vi "CTRE_Phoenix_MotorControl_ConfigureAllSettings.vi"(6 "timeoutMs":i32=50, 7 "Force Write":bool, 8 "error in (no error)":errorcluster, 10 "Motor Controller Configurables":T1={"Base Configurables"={"openLoopRamp"=0.0, "closedLoopRamp"=0.0, "peakOutputForward"=1.0, "peakOutputReverse"=-1.0, "nominalOutputForward"=0.0, "nominalOutputReverse"=0.0, "neutralDeadband"=0.04, "voltageCompSaturation"=0.0, "voltageMeasurementFilter"=32, "velocityMeasurementPeriod"=100, "velocityMeasurementWindow"=64, "forwardSoftLimitThreshold"=0, "reverseSoftLimitThreshold"=0, "forwardSoftLimitEnable"=FALSE, "reverseSoftLimitEnable"=FALSE, "slot0"={"P"=0.0, "I"=0.0, "D"=0.0, "F"=0.0, "integralZone"=0.0, "allowableClosedLoopError"=0, "maxIntegralAccumulator"=0.0, "closedLoopPeakOutput"=1.0, "closedLoopPeriod"=1}, "slot1"={"P"=0.0, "I"=0.0, "D"=0.0, "F"=0.0, "integralZone"=0.0, "allowableClosedLoopError"=0, "maxIntegralAccumulator"=0.0, "closedLoopPeakOutput"=1.0, "closedLoopPeriod"=1}, "slot2"={"P"=0.0, "I"=0.0, "D"=0.0, "F"=0.0, "integralZone"=0.0, "allowableClosedLoopError"=0, "maxIntegralAccumulator"=0.0, "closedLoopPeakOutput"=1.0, "closedLoopPeriod"=1}, "slot3"={"P"=0.0, "I"=0.0, "D"=0.0, "F"=0.0, "integralZone"=0.0, "allowableClosedLoopError"=0, "maxIntegralAccumulator"=0.0, "closedLoopPeakOutput"=1.0, "closedLoopPeriod"=1}, "auxPIDPolarity"=FALSE, "remoteFilter0"={"remoteSensorDeviceID"=0, "remoteSensorSource"=enum."Off"}, "remoteFilter1"={"remoteSensorDeviceID"=0, "remoteSensorSource"=enum."Off"}, "motionCruiseVelocity"=0, "motionAcceleration"=0, "motionProfileTrajectoryPeriod"=0, "feedbackNotContinuous"=FALSE, "remoteSensorClosedLoopDisableNeutralOnLOS"=FALSE, "clearPositionOnLimitF"=FALSE, "clearPositionOnLimitR"=FALSE, "clearPositionOnQuadIdx"=FALSE, "limitSwitchDisableNeutralOnLOS"=FALSE, "softLimitDisableNeutralOnLOS"=FALSE, "pulseWidthPeriod_EdgesPerRot"=1, "pulseWidthPeriod_FilterWindowSz"=1, "customParam"={"customParam0"=0, "customParam1"=0}, "trajectoryInterpolationEnable"=TRUE}, "primaryPID"={"selectedFeedbackCoefficient"=1.0, "selectedFeedbackSensor"=11}, "auxiliaryPID"={"selectedFeedbackCoefficient"=1.0, "selectedFeedbackSensor"=11}, "sum 0 term"=11, "sum 1 term"=11, "diff 0 term "=11, "diff 1 term"=11, "forwardLimitSwitchDeviceID"=0, "reverseLimitSwitchDeviceID"=0, "forwardLimitSwitchNormal"=enum."Normally Open", "reverseLimitSwitchNormal"=enum."Normally Open", "forwardLimitSwitchSource"=3, "reverseLimitSwitchSource"=3} {"diff 1 term" items=["Remote Source 0"=11, "Remote Source 1"=12, "Software Emulated"=15]; "diff 0 term" items=["Remote Source 0"=11, "Remote Source 1"=12, "Software Emulated"=15]; "sum 1 term" items=["Remote Source 0"=11, "Remote Source 1"=12, "Software Emulated"=15]; "sum 0 term" items=["Remote Source 0"=11, "Remote Source 1"=12, "Software Emulated"=15]; "reverseLimitSwitchSource" items=["Remote Talon SRX"=1, "Remote CANifier"=2, "Deactivated"=3]; "forwardLimitSwitchSource" items=["Remote Talon SRX"=1, "Remote CANifier"=2, "Deactivated"=3]; "auxiliaryPID"."selectedFeedbackSensor" items=["Sensor Sum (S0 + S1)"=9, "Sensor Difference (D0 - D1)"=10, "Remote Source 0"=11, "Remote Source 1"=12, "Software Emulated"=15]; "primaryPID"."selectedFeedbackSensor" items=["Sensor Sum (S0 + S1)"=9, "Sensor Difference (D0 - D1)"=10, "Remote Source 0"=11, "Remote Source 1"=12, "Software Emulated"=15]; "Base Configurables"."velocityMeasurementPeriod" items=["Period_1ms"=1, "Period_2ms"=2, "Period_5ms"=5, "Period_10ms"=10, "Period_20ms"=20, "Period_25ms"=25, "Period_50ms"=50, "Period_100ms"=100]}, 11 "PhoenixMotorControlDevRef":T12={"DeviceStatus"={"status"=FALSE, "code"=0, "source"=""}, "Type"=enum."PWM", "PWM"={"PWM Channel"=enum."PWM 1", "DeadBand"={"Name"="", "maxPositivePwm"=0, "minPositivePwm"=0, "centerPwm"=0, "maxNegativePwm"=0, "minNegativePwm"=0, "angularRange"=0}}, "CAN"={"Device Number"=0, "SetOutput VI Ref"=variant(enum8{"Percent VBus", "Current", "Speed", "Position", "Voltage"} enum."Percent VBus"), "GetOutput VI Ref"=variant(refnum<k1> refnum), "Enable VI Ref"=variant(dbl 12.0), "Disable VI Ref"=variant(enum8{"Percent VBus", "Speed", "Position", "Slave", "Unchanged / Invalid", "Voltage Compensation", "Current", "Motion Profile"} enum."Percent VBus"), "Data"=variant}, "Invert"=FALSE, "DIO PWM"={"PWM \"Enable\" Channel"=enum."Invalid", "DIOChannel"=enum."Invalid", "PWM Rate"=0.0}}) -> (0 "error out":errorcluster, 3 "PhoenixMotorControlDevRef":T12={"DeviceStatus"={"status"=FALSE, "code"=0, "source"=""}, "Type"=enum."PWM", "PWM"={"PWM Channel"=enum."PWM 1", "DeadBand"={"Name"="", "maxPositivePwm"=0, "minPositivePwm"=0, "centerPwm"=0, "maxNegativePwm"=0, "minNegativePwm"=0, "angularRange"=0}}, "CAN"={"Device Number"=0, "SetOutput VI Ref"=variant(enum8{"Percent VBus", "Current", "Speed", "Position", "Voltage"} enum."Percent VBus"), "GetOutput VI Ref"=variant(refnum<k1> refnum), "Enable VI Ref"=variant(dbl 12.0), "Disable VI Ref"=variant(enum8{"Percent VBus", "Speed", "Position", "Slave", "Unchanged / Invalid", "Voltage Compensation", "Current", "Motion Profile"} enum."Percent VBus"), "Data"=variant}, "Invert"=FALSE, "DIO PWM"={"PWM \"Enable\" Channel"=enum."Invalid", "DIOChannel"=enum."Invalid", "PWM Rate"=0.0}})   [LabVIEW 2020]
doc: "Configures all persistant settings\n\n<b> Motor Controller Configurables </b> Cluster of all items to be configured"
uses:
  <vilib>/Rock Robotics/WPI/MotorControl/WPI_MotorControlDeviceRef.ctl
  <vilib>/Rock Robotics/WPI/MotorControl/WPI_MotorControlType.ctl
  <vilib>/Rock Robotics/SystemInterfaces/DIO/FPGA_DIOPWMChannel.ctl
  <vilib>/Rock Robotics/WPI/PWM/WPI_PWMDeadband.ctl
  <vilib>/Rock Robotics/SystemInterfaces/DIO/FPGA_DIOChannel.ctl
  <vilib>/Rock Robotics/WPI/ThirdParty/Phoenix-LabVIEW/Motor Controller/Controls/CTRE_Phoenix_MotorControl_MotorControllerConfigurables.ctl
  <vilib>/Rock Robotics/WPI/ThirdParty/Phoenix-LabVIEW/Motor Controller/Controls/CTRE_Phoenix_MotorControl_BaseConfigurables.ctl
  <vilib>/Rock Robotics/WPI/ThirdParty/Phoenix-LabVIEW/Motor Controller/Controls/CTRE_Phoenix_MotorControl_VelocityMeasurementPeriod.ctl
  <vilib>/Rock Robotics/WPI/ThirdParty/Phoenix-LabVIEW/Motor Controller/Controls/CTRE_Phoenix_MotorControl_SlotStructure.ctl
  <vilib>/Rock Robotics/WPI/ThirdParty/Phoenix-LabVIEW/Motor Controller/Controls/CTRE_Phoenix_MotorControl_FilterStruct.ctl
  <vilib>/Rock Robotics/WPI/ThirdParty/Phoenix-LabVIEW/Motor Controller/Controls/CTRE_Phoenix_MotorControl_RemoteSourceType.ctl
  <vilib>/Rock Robotics/WPI/ThirdParty/Phoenix-LabVIEW/Controls/CTRE_Phoenix_CustomParamConfiguration.ctl
  <vilib>/Rock Robotics/WPI/ThirdParty/Phoenix-LabVIEW/Motor Controller/Controls/CTRE_Phoenix_MotorControl_RemoteFeedbackDevice.ctl
  <vilib>/Rock Robotics/WPI/ThirdParty/Phoenix-LabVIEW/Motor Controller/Controls/CTRE_Phoenix_MotorControl_SensorTermFeedbackDevice.ctl
  <vilib>/Rock Robotics/WPI/ThirdParty/Phoenix-LabVIEW/Motor Controller/Controls/CTRE_Phoenix_MotorControl_LimitSwitchNormal.ctl
  <vilib>/Rock Robotics/WPI/ThirdParty/Phoenix-LabVIEW/Motor Controller/Controls/CTRE_Phoenix_MotorControl_LimitSwitchSource.ctl
panel:
  # "Sum and Diff terms are ways to select more than one sensor as a feedback device. \n Sum 0 is the first feedback device to be used for the Sum term, \n Sum 1 is the feedback device to be added to Sum 0 for the Sum term\n Diff 0 and Diff 1 work in a similar manner"
  # "These are only applicable\nif using a remote limit switch.\n\nLocal limit switches/no limit\nswitches do not use this"
  # "False: Primary Output = PID[0] + PID[1]  ---  Auxiliary Output = PID[0] - PID[1]\nTrue:  Primary Output = PID[0] - PID[1] --- Auxiliary Output = PID[0] + PID[1]"
  # "Enable the motion profile executor to perform linear interpolation between profile points.  Defaults to True."
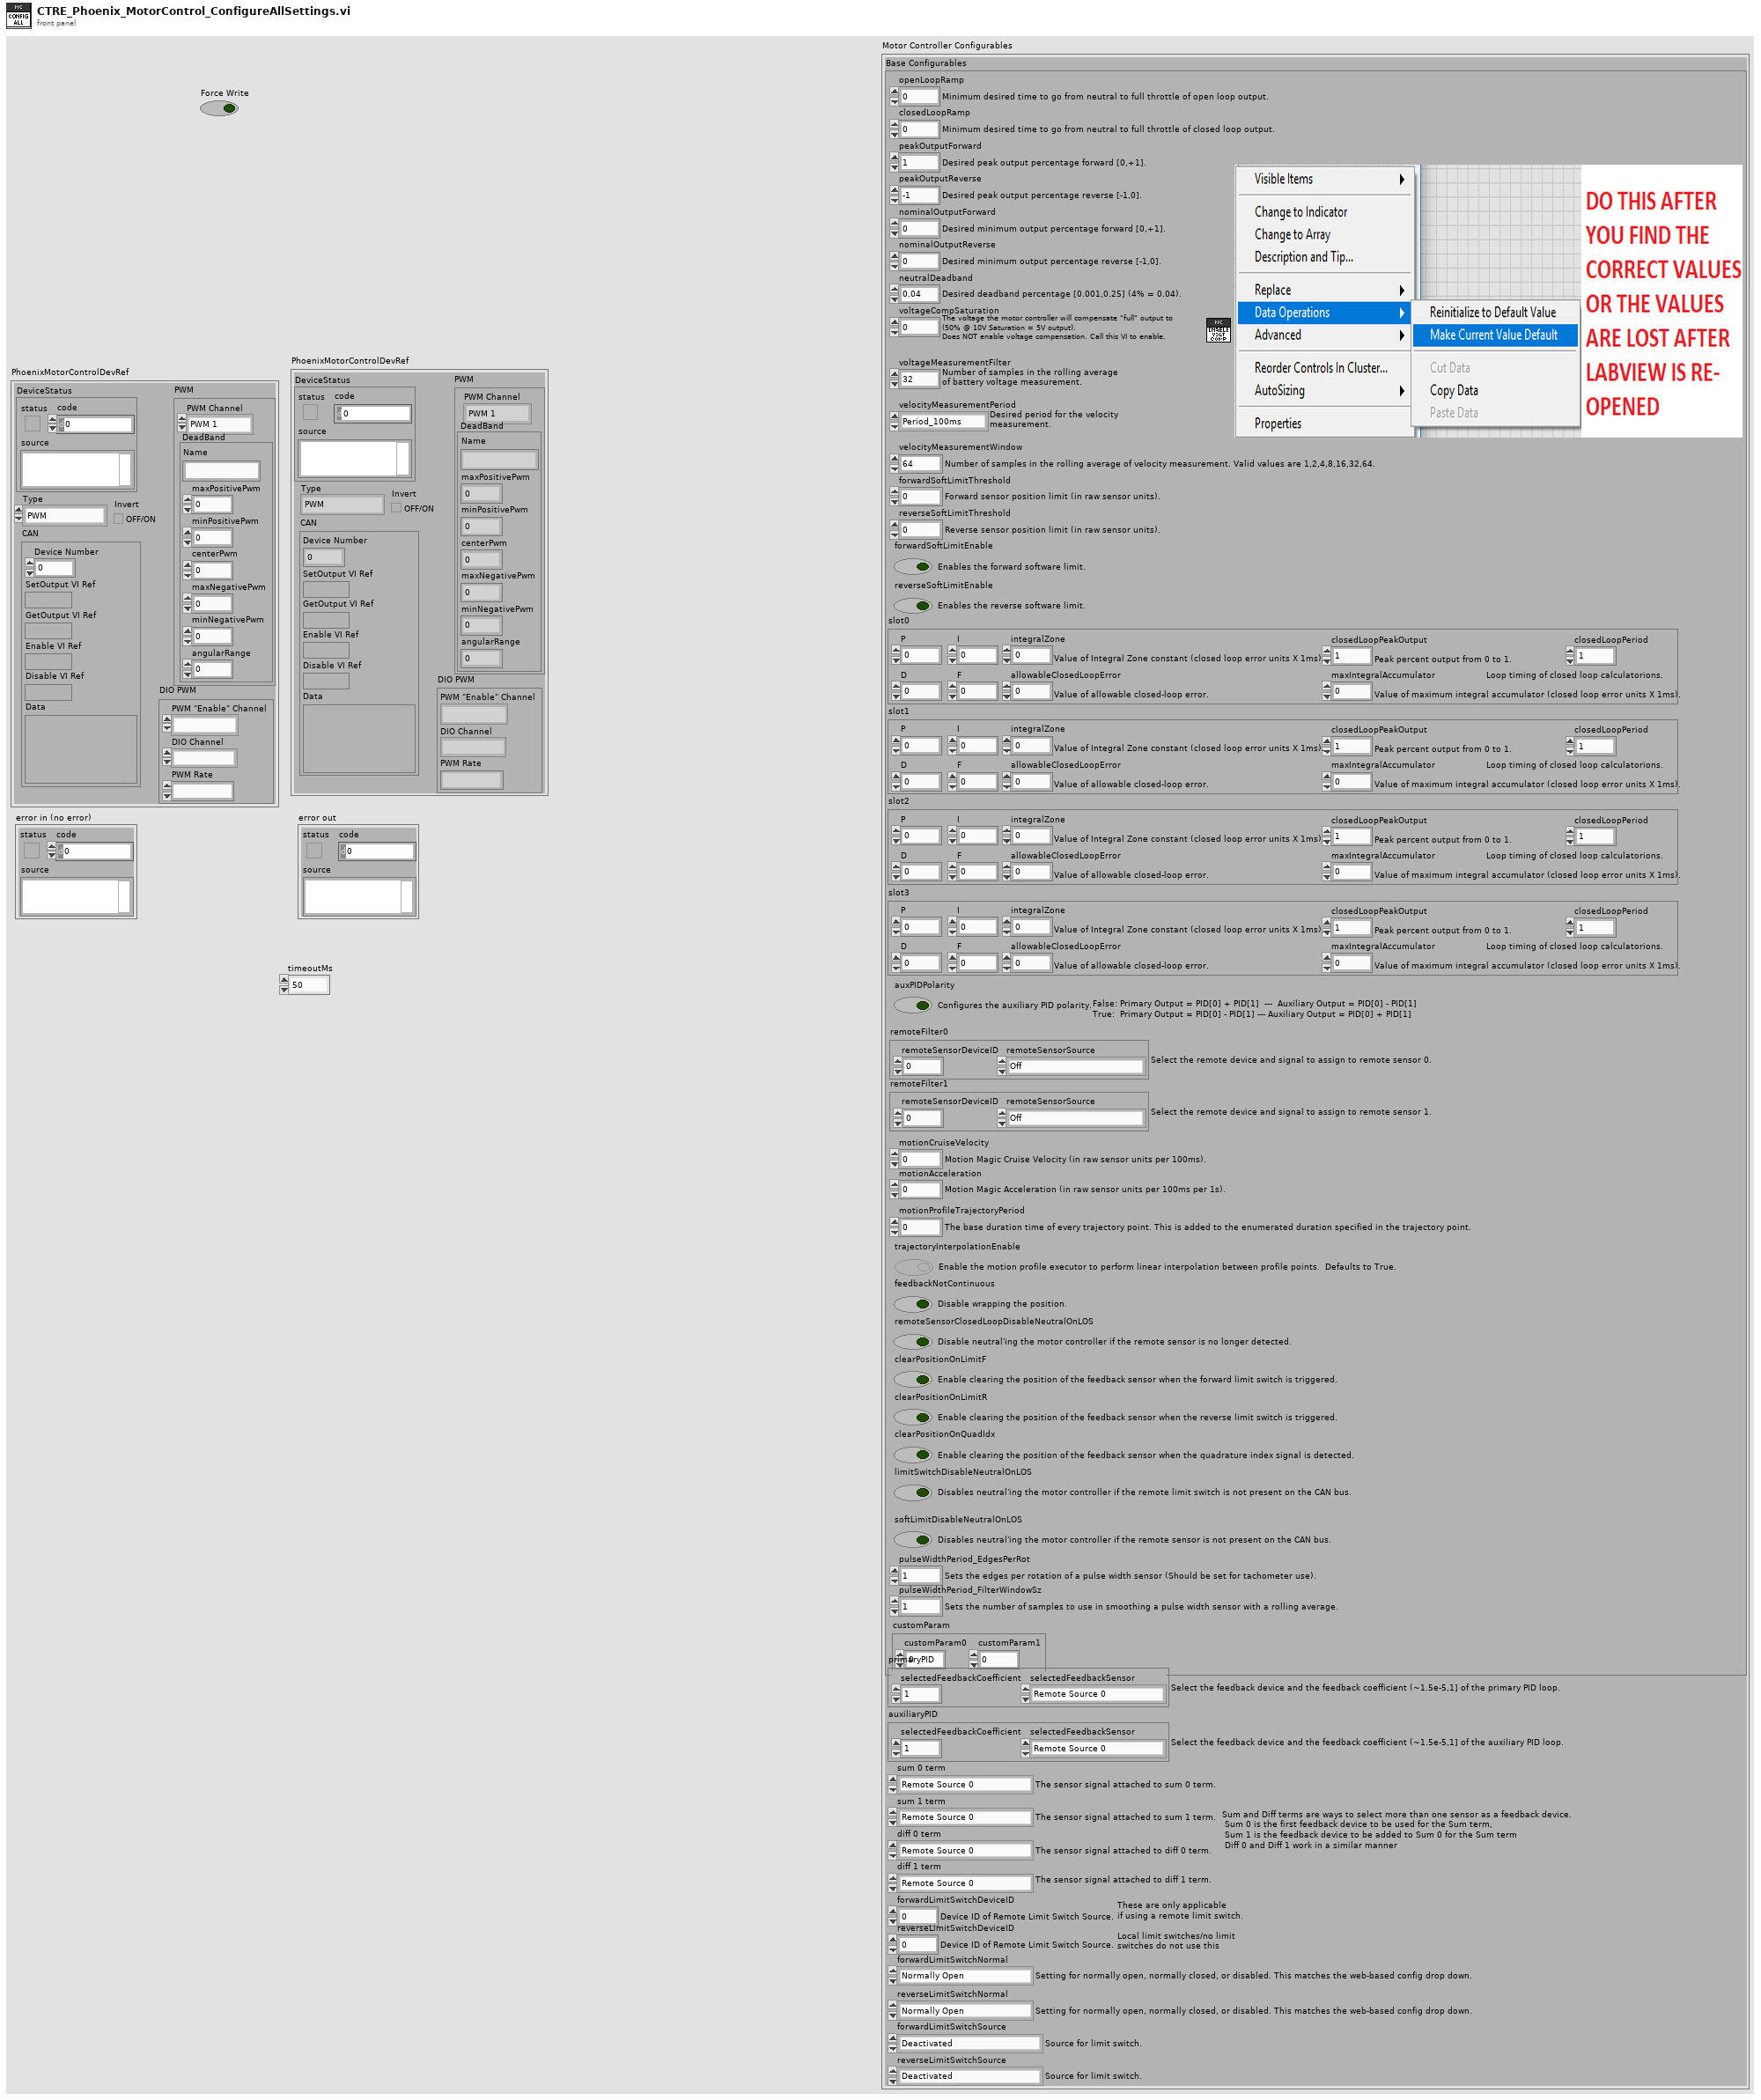
[diagram p1: front panel]
types:
  T1 = typedef "CTRE_Phoenix_MotorControl_MotorControllerConfigurables.ctl" = cluster{"Base Configurables":T2, "primaryPID":cluster{"selectedFeedbackCoefficient":dbl, "selectedFeedbackSensor":T8}, "auxiliaryPID":cluster{"selectedFeedbackCoefficient":dbl, "selectedFeedbackSensor":T8}, "sum 0 term":T9, "sum 1 term":T9, "diff 0 term ":T9, "diff 1 term":T9, "forwardLimitSwitchDeviceID":i32, "reverseLimitSwitchDeviceID":i32, "forwardLimitSwitchNormal":T10, "reverseLimitSwitchNormal":T10, "forwardLimitSwitchSource":T11, "reverseLimitSwitchSource":T11}
  T2 = typedef "CTRE_Phoenix_MotorControl_BaseConfigurables.ctl" = cluster{"openLoopRamp":dbl, "closedLoopRamp":dbl, "peakOutputForward":dbl, "peakOutputReverse":dbl, "nominalOutputForward":dbl, "nominalOutputReverse":dbl, "neutralDeadband":dbl, "voltageCompSaturation":dbl, "voltageMeasurementFilter":i32, "velocityMeasurementPeriod":T3, "velocityMeasurementWindow":i32, "forwardSoftLimitThreshold":i32, "reverseSoftLimitThreshold":i32, "forwardSoftLimitEnable":bool, "reverseSoftLimitEnable":bool, "slot0":T4, "slot1":T4, "slot2":T4, "slot3":T4, "auxPIDPolarity":bool, "remoteFilter0":T5, "remoteFilter1":T5, "motionCruiseVelocity":i32, "motionAcceleration":i32, "motionProfileTrajectoryPeriod":i32, "feedbackNotContinuous":bool, "remoteSensorClosedLoopDisableNeutralOnLOS":bool, "clearPositionOnLimitF":bool, "clearPositionOnLimitR":bool, "clearPositionOnQuadIdx":bool, "limitSwitchDisableNeutralOnLOS":bool, "softLimitDisableNeutralOnLOS":bool, "pulseWidthPeriod_EdgesPerRot":i32, "pulseWidthPeriod_FilterWindowSz":i32, "customParam":T7, "trajectoryInterpolationEnable":bool}
  T3 = typedef "CTRE_Phoenix_MotorControl_VelocityMeasurementPeriod.ctl" = u16
  T4 = typedef "CTRE_Phoenix_MotorControl_SlotStructure.ctl" = cluster{"P":dbl, "I":dbl, "D":dbl, "F":dbl, "integralZone":dbl, "allowableClosedLoopError":i32, "maxIntegralAccumulator":dbl, "closedLoopPeakOutput":dbl, "closedLoopPeriod":i32}
  T5 = typedef "CTRE_Phoenix_MotorControl_FilterStruct.ctl" = cluster{"remoteSensorDeviceID":u8, "remoteSensorSource":T6}
  T6 = typedef "CTRE_Phoenix_MotorControl_RemoteSourceType.ctl" = enum16{"Off", "Talon SRX Selected Sensor", "Pigeon IMU Yaw", "Pigeon IMU Pitch", "Pigeon IMU Roll", "CANifier Quadrature", "CANifier PWM Input 0", "CANifier PWM Input 1", "CANifier PWM Input 2", "CANifier PWM Input 3", "Gadgeteer Pigeon Yaw", "Gadgeteer Pigeon Pitch", "Gadgeteer Pigeon Roll", "CANCoder"}
  T7 = typedef "CTRE_Phoenix_CustomParamConfiguration.ctl" = cluster{"customParam0":i32, "customParam1":i32}
  T8 = typedef "CTRE_Phoenix_MotorControl_RemoteFeedbackDevice.ctl" = i8
  T9 = typedef "CTRE_Phoenix_MotorControl_SensorTermFeedbackDevice.ctl" = i8
  T10 = typedef "CTRE_Phoenix_MotorControl_LimitSwitchNormal.ctl" = enum16{"Normally Open", "Normally Closed", "Disabled"}
  T11 = typedef "CTRE_Phoenix_MotorControl_LimitSwitchSource.ctl" = u16
  T12 = typedef "WPI_MotorControlDeviceRef.ctl" = cluster{"DeviceStatus":errorcluster, "Type":T13, "PWM":cluster{"PWM Channel":T14, "DeadBand":T15}, "CAN":cluster{"Device Number":u8, "SetOutput VI Ref":variant, "GetOutput VI Ref":variant, "Enable VI Ref":variant, "Disable VI Ref":variant, "Data":variant}, "Invert":bool, "DIO PWM":cluster{"PWM \"Enable\" Channel":T14, "DIOChannel":T16, "PWM Rate":dbl}}
  T13 = typedef "WPI_MotorControlType.ctl" = enum16{"PWM", "CAN", "DIO PWM"}
  T14 = typedef "FPGA_DIOPWMChannel.ctl" = enum8{"PWM 0", "PWM 1", "PWM 2", "PWM 3", "PWM 4", "PWM 5", "PWM 6", "PWM 7", "PWM 8", "PWM 9", "PWM MXP 0", "PWM MXP 1", "PWM MXP 2", "PWM MXP 3", "PWM MXP 4", "PWM MXP 5", "PWM MXP 6", "PWM MXP 7", "PWM MXP 8", "PWM MXP 9", "Invalid"}
  T15 = typedef "WPI_PWMDeadband.ctl" = cluster{"Name":string, "maxPositivePwm":i32, "minPositivePwm":i32, "centerPwm":i32, "maxNegativePwm":i32, "minNegativePwm":i32, "angularRange":u16}
  T16 = typedef "FPGA_DIOChannel.ctl" = enum8{"DIO 0", "DIO 1", "DIO 2", "DIO 3", "DIO 4", "DIO 5", "DIO 6", "DIO 7", "DIO 8", "DIO 9", "DIO MXP 0", "DIO MXP 1", "DIO MXP 2", "DIO MXP 3", "DIO MXP 4", "DIO MXP 5", "DIO MXP 6", "DIO MXP 7", "DIO MXP 8", "DIO MXP 9", "DIO MXP 10", "DIO MXP 11", "DIO MXP 12", "DIO MXP 13", "DIO MXP 14", "DIO MXP 15", "SPI Port CS1", "SPI Port CS2", "SPI Port CS3", "SPI Port MISO", "SPI Port MOSI", "Invalid"}
  T17 = cluster{"Base Configurables":cluster{"openLoopRamp":bool, "closedLoopRamp":bool, "peakOutputForward":bool, "peakOutputReverse":bool, "nominalOutputForward":bool, "nominalOutputReverse":bool, "neutralDeadband":bool, "voltageCompSaturation":bool, "voltageMeasurementFilter":bool, "velocityMeasurementPeriod":bool, "velocityMeasurementWindow":bool, "forwardSoftLimitThreshold":bool, "reverseSoftLimitThreshold":bool, "forwardSoftLimitEnable":bool, "reverseSoftLimitEnable":bool, "slot0":cluster{"P":bool, "I":bool, "D":bool, "F":bool, "integralZone":bool, "allowableClosedLoopError":bool, "maxIntegralAccumulator":bool, "closedLoopPeakOutput":bool, "closedLoopPeriod":bool}, "slot1":cluster{"P":bool, "I":bool, "D":bool, "F":bool, "integralZone":bool, "allowableClosedLoopError":bool, "maxIntegralAccumulator":bool, "closedLoopPeakOutput":bool, "closedLoopPeriod":bool}, "slot2":cluster{"P":bool, "I":bool, "D":bool, "F":bool, "integralZone":bool, "allowableClosedLoopError":bool, "maxIntegralAccumulator":bool, "closedLoopPeakOutput":bool, "closedLoopPeriod":bool}, "slot3":cluster{"P":bool, "I":bool, "D":bool, "F":bool, "integralZone":bool, "allowableClosedLoopError":bool, "maxIntegralAccumulator":bool, "closedLoopPeakOutput":bool, "closedLoopPeriod":bool}, "auxPIDPolarity":bool, "remoteFilter0":cluster{"remoteSensorDeviceID":bool, "remoteSensorSource":bool}, "remoteFilter1":cluster{"remoteSensorDeviceID":bool, "remoteSensorSource":bool}, "motionCruiseVelocity":bool, "motionAcceleration":bool, "motionProfileTrajectoryPeriod":bool, "feedbackNotContinuous":bool, "remoteSensorClosedLoopDisableNeutralOnLOS":bool, "clearPositionOnLimitF":bool, "clearPositionOnLimitR":bool, "clearPositionOnQuadIdx":bool, "limitSwitchDisableNeutralOnLOS":bool, "softLimitDisableNeutralOnLOS":bool, "pulseWidthPeriod_EdgesPerRot":bool, "pulseWidthPeriod_FilterWindowSz":bool, "customParam":cluster{"customParam0":bool, "customParam1":bool}, "trajectoryInterpolationEnable":bool}, "primaryPID":cluster{"selectedFeedbackCoefficient":bool, "selectedFeedbackSensor":bool}, "auxiliaryPID":cluster{"selectedFeedbackCoefficient":bool, "selectedFeedbackSensor":bool}, "sum 0 term":bool, "sum 1 term":bool, "diff 0 term ":bool, "diff 1 term":bool, "forwardLimitSwitchDeviceID":bool, "reverseLimitSwitchDeviceID":bool, "forwardLimitSwitchNormal":bool, "reverseLimitSwitchNormal":bool, "forwardLimitSwitchSource":bool, "reverseLimitSwitchSource":bool}
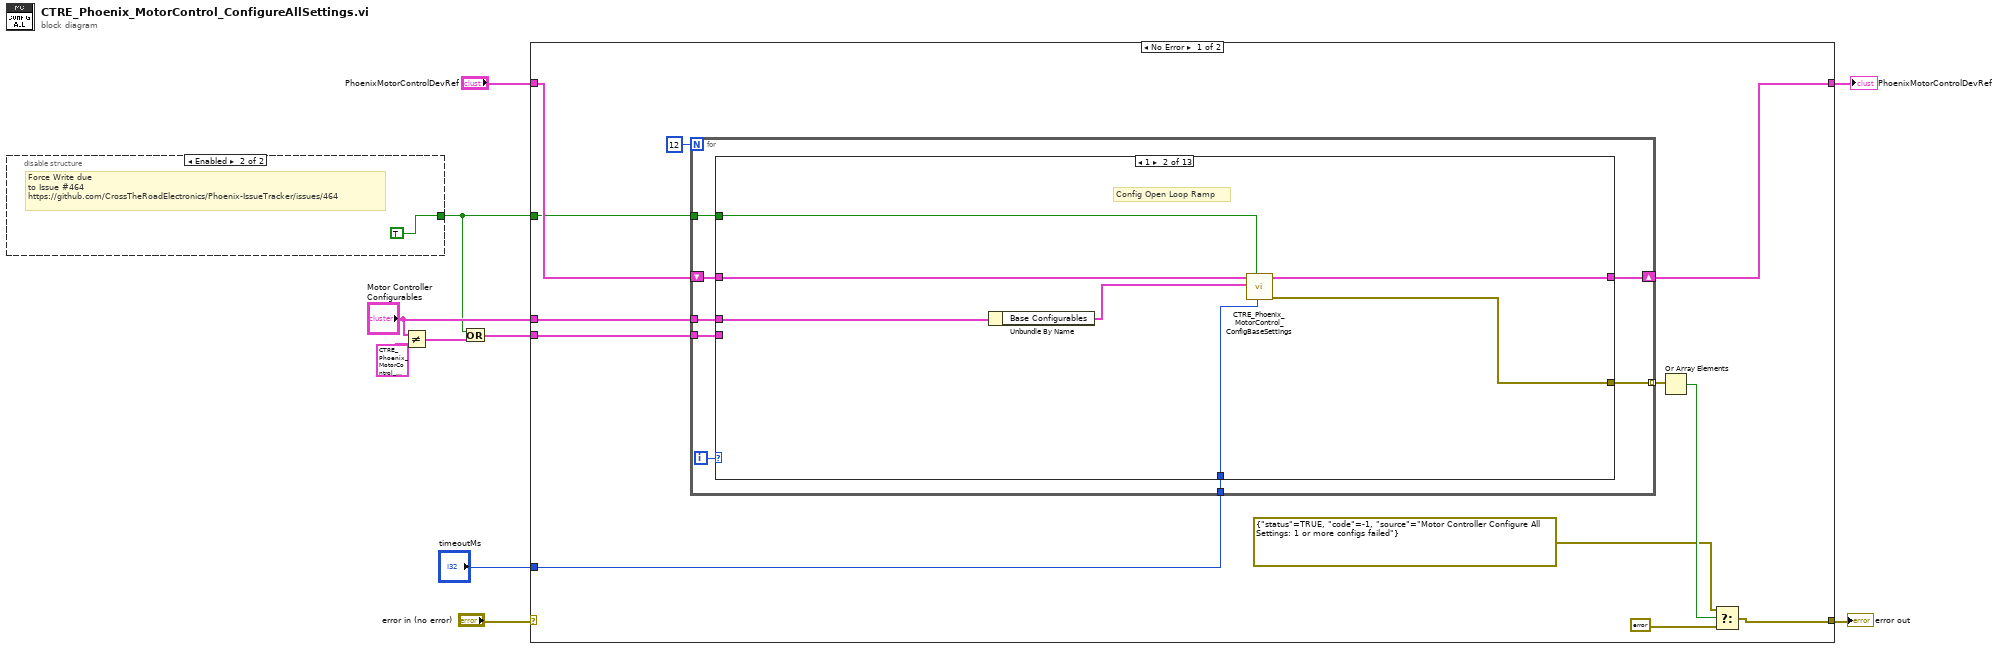
[diagram p0: block diagram]
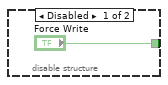
[diagram p2: hidden frame]
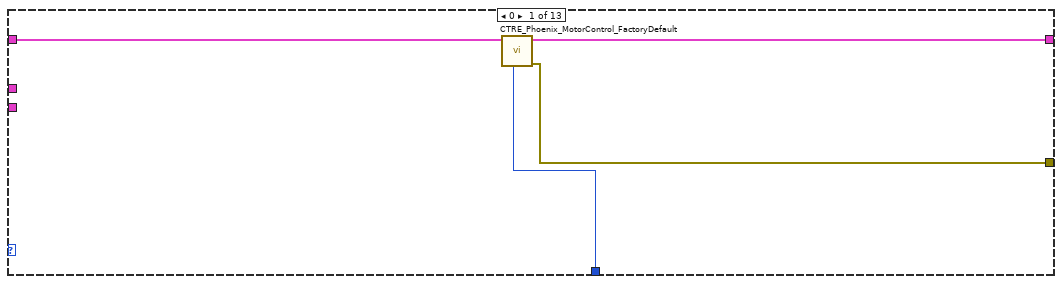
[diagram p3: hidden frame]
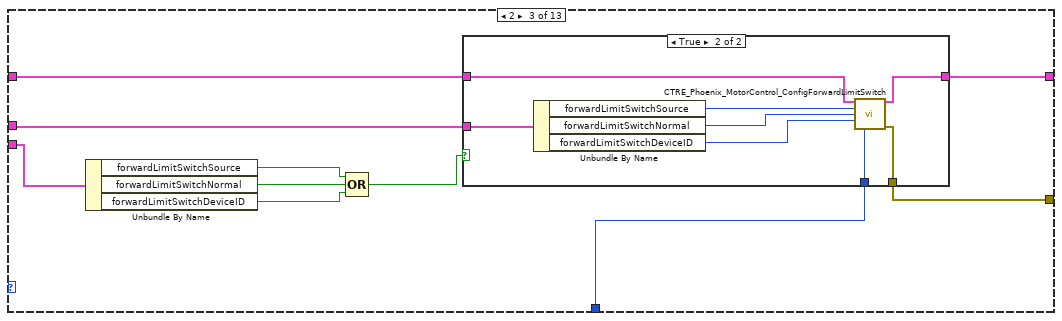
[diagram p4: hidden frame]
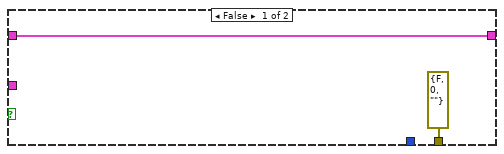
[diagram p5: hidden frame]
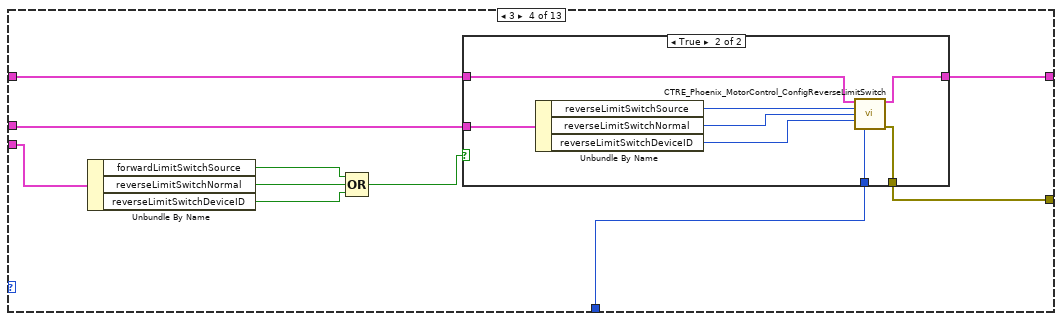
[diagram p6: hidden frame]
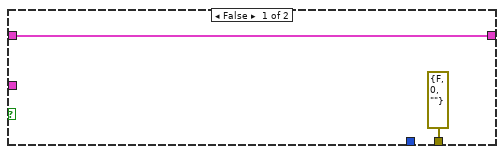
[diagram p7: hidden frame]
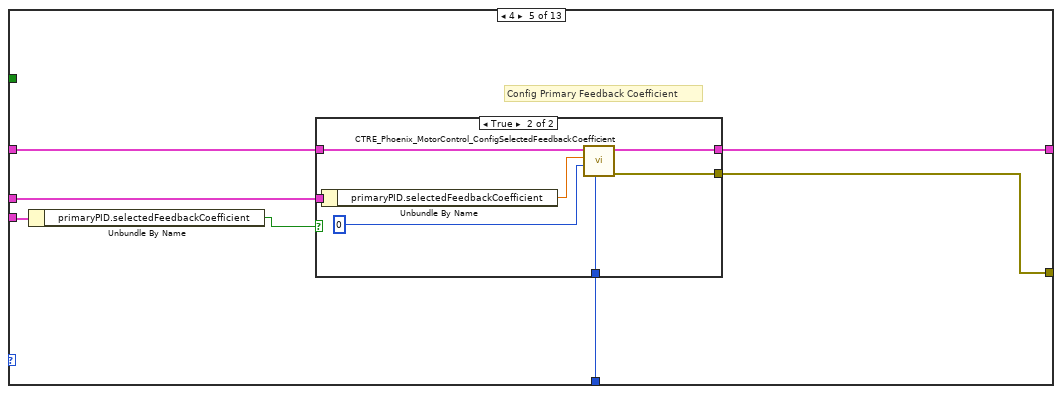
[diagram p8: hidden frame]
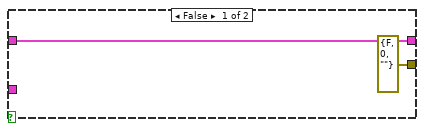
[diagram p9: hidden frame]
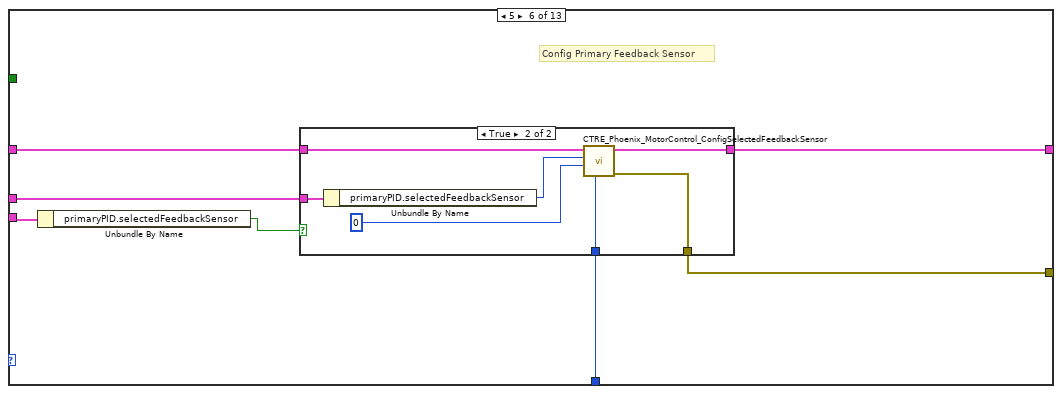
[diagram p10: hidden frame]
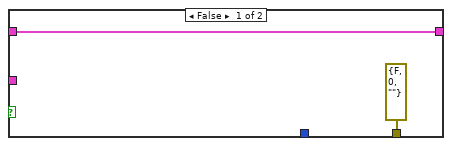
[diagram p11: hidden frame]
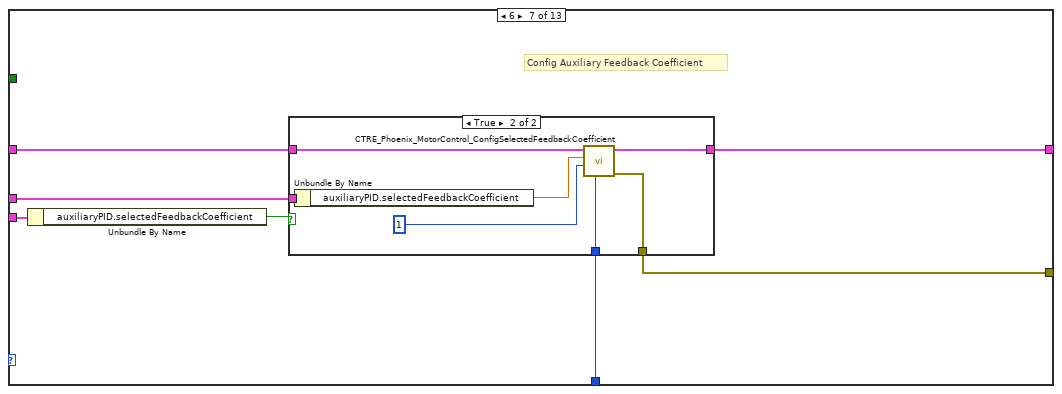
[diagram p12: hidden frame]
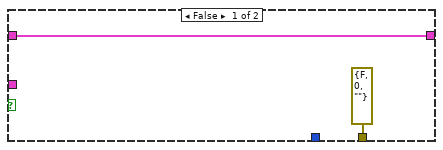
[diagram p13: hidden frame]
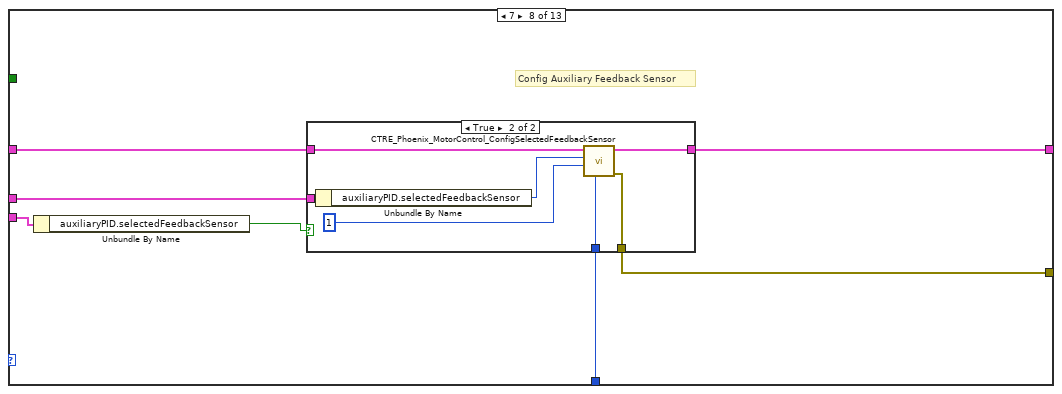
[diagram p14: hidden frame]
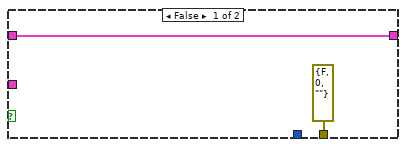
[diagram p15: hidden frame]
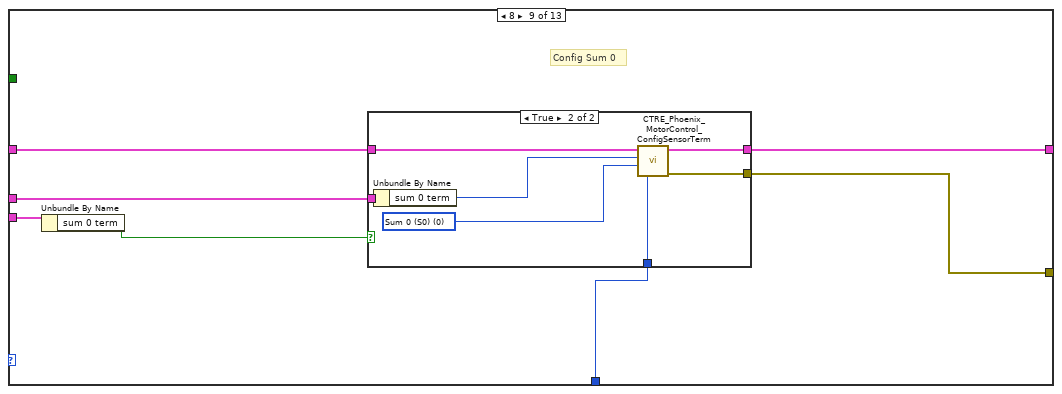
[diagram p16: hidden frame]
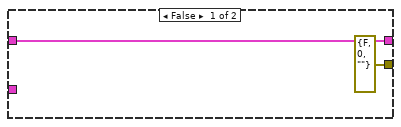
[diagram p17: hidden frame]
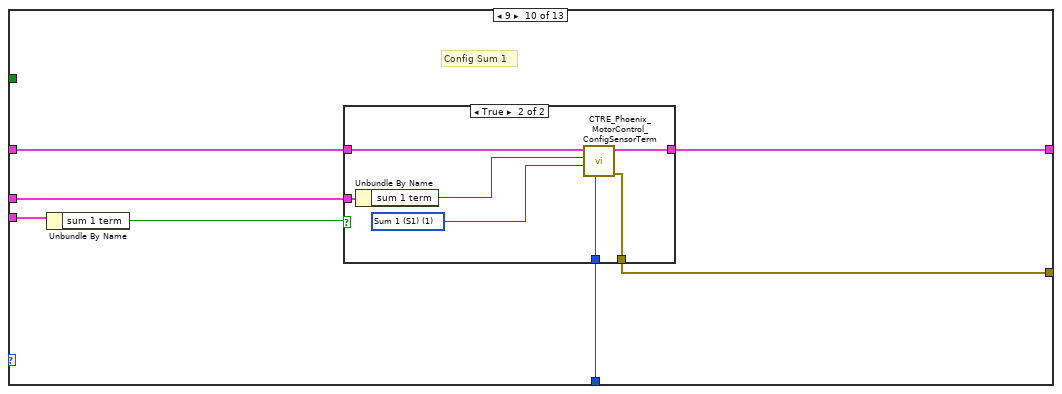
[diagram p18: hidden frame]
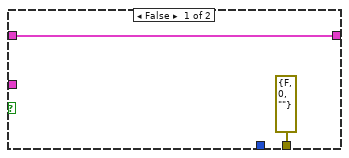
[diagram p19: hidden frame]
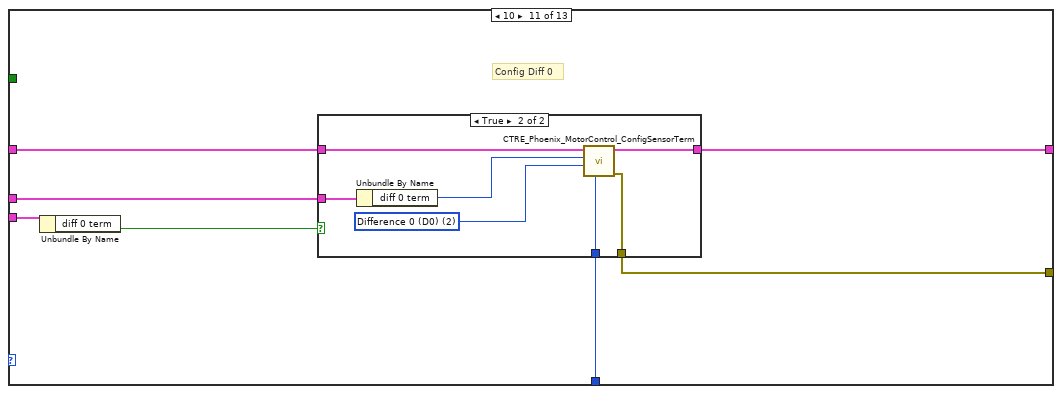
[diagram p20: hidden frame]
diagram:
  n1 = disable-structure shown="Enabled" {
    disable-tunnel: ["Force Write" TRUE ("Force Write")] -> w1
    frame Disabled {
    }
    frame Enabled {
      # "Force Write due\nto Issue #464\nhttps://github.com/CrossTheRoadElectronics/Phoenix-IssueTracker/issues/464"
    }
  }
  n2 = Not Equal?(x="Motor Controller Configurables", y=T1 {"Base Configurables"={"openLoopRamp"=0.0, "closedLoopRamp"=0.0, "peakOutputForward"=1.0, "peakOutputReverse"=-1.0, "nominalOutputForward"=0.0, "nominalOutputReverse"=0.0, "neutralDeadband"=0.04, "voltageCompSaturation"=0.0, "voltageMeasurementFilter"=32, "velocityMeasurementPeriod"=100, "velocityMeasurementWindow"=64, "forwardSoftLimitThreshold"=0, "reverseSoftLimitThreshold"=0, "forwardSoftLimitEnable"=FALSE, "reverseSoftLimitEnable"=FALSE, "slot0"={"P"=0.0, "I"=0.0, "D"=0.0, "F"=0.0, "integralZone"=0.0, "allowableClosedLoopError"=0, "maxIntegralAccumulator"=0.0, "closedLoopPeakOutput"=1.0, "closedLoopPeriod"=1}, "slot1"={"P"=0.0, "I"=0.0, "D"=0.0, "F"=0.0, "integralZone"=0.0, "allowableClosedLoopError"=0, "maxIntegralAccumulator"=0.0, "closedLoopPeakOutput"=1.0, "closedLoopPeriod"=1}, "slot2"={"P"=0.0, "I"=0.0, "D"=0.0, "F"=0.0, "integralZone"=0.0, "allowableClosedLoopError"=0, "maxIntegralAccumulator"=0.0, "closedLoopPeakOutput"=1.0, "closedLoopPeriod"=1}, "slot3"={"P"=0.0, "I"=0.0, "D"=0.0, "F"=0.0, "integralZone"=0.0, "allowableClosedLoopError"=0, "maxIntegralAccumulator"=0.0, "closedLoopPeakOutput"=1.0, "closedLoopPeriod"=1}, "auxPIDPolarity"=FALSE, "remoteFilter0"={"remoteSensorDeviceID"=0, "remoteSensorSource"=enum."Off"}, "remoteFilter1"={"remoteSensorDeviceID"=0, "remoteSensorSource"=enum."Off"}, "motionCruiseVelocity"=0, "motionAcceleration"=0, "motionProfileTrajectoryPeriod"=0, "feedbackNotContinuous"=FALSE, "remoteSensorClosedLoopDisableNeutralOnLOS"=FALSE, "clearPositionOnLimitF"=FALSE, "clearPositionOnLimitR"=FALSE, "clearPositionOnQuadIdx"=FALSE, "limitSwitchDisableNeutralOnLOS"=FALSE, "softLimitDisableNeutralOnLOS"=FALSE, "pulseWidthPeriod_EdgesPerRot"=1, "pulseWidthPeriod_FilterWindowSz"=1, "customParam"={"customParam0"=0, "customParam1"=0}, "trajectoryInterpolationEnable"=TRUE}, "primaryPID"={"selectedFeedbackCoefficient"=1.0, "selectedFeedbackSensor"=11}, "auxiliaryPID"={"selectedFeedbackCoefficient"=1.0, "selectedFeedbackSensor"=11}, "sum 0 term"=11, "sum 1 term"=11, "diff 0 term "=11, "diff 1 term"=11, "forwardLimitSwitchDeviceID"=0, "reverseLimitSwitchDeviceID"=0, "forwardLimitSwitchNormal"=enum."Normally Open", "reverseLimitSwitchNormal"=enum."Normally Open", "forwardLimitSwitchSource"=3, "reverseLimitSwitchSource"=3}) -> (x != y?=w3:T17)
  n3 = Or(x=w1, y=w3) -> (x .or. y?=w2:T17)
  n4 = case shown="No Error" "error in (no error)" {
    selector: "error in (no error)" -> [_ w215]
    tunnel: [w20 w215] -> w10
    tunnel: "PhoenixMotorControlDevRef" -> [w24 w214]
    tunnel: [w23 w214] -> w8
    tunnel: "timeoutMs" -> [w22 _]
    tunnel: "Motor Controller Configurables" -> [w21 _]
    tunnel: w2 -> [w14 _]
    tunnel: w1 -> [w13 _]
    frame No Error {
      n5 = for {
        N: 12 -> [_]
        tunnel: w22 -> [w30]
        tunnel: w21 -> [w29]
        shift-right: [w31] -> w23
        shift-left: w24 -> [w32]
        tunnel: [w27] -> w16 mode=indexing
        tunnel: w14 -> [w26]
        tunnel: w13 -> [w25]
        i -> [w28]
        n6 = case shown="1" w28 {
          tunnel: w32 -> [w36 w42 w52 w72 w89 w105 w122 w134 w152 w169 w182 w199 w213]
          tunnel: [w35 w39 w51 w71 w88 w106 w121 w135 w153 w167 w185 w200 w213] -> w31
          tunnel: w30 -> [w33 w40 w49 w69 w86 w104 w120 w137 w151 w168 w183 w201 _]
          tunnel: w29 -> [_ w43 w53 w73 w90 w102 w118 w138 w154 w170 w186 w202 _]
          tunnel: [w34 w37 w50 w70 w87 w103 w119 w136 w150 w166 w184 w198 errorcluster {"status"=FALSE, "code"=0, "source"=""} ("error out")] -> w27
          tunnel: w26 -> [_ _ w48 w68 w85 w101 w117 w133 w149 w165 w181 w197 _]
          tunnel: w25 -> [_ w38 _ _ _ _ _ _ _ _ _ _ _]
          frame 0 {
            n7 = call <vilib>:"CTRE_Phoenix_MotorControl_FactoryDefault.vi"("timeoutMs"=w33, "PhoenixMotorControlDevRef"=w36) -> ("error out"=w34:errorcluster, "PhoenixMotorControlDevRef"=w35:T12)  [unwired: 8 in]
          }
          frame 1 {
            # "Config Open Loop Ramp"
            n8 = Unbundle By Name(w43) -> ("Base Configurables"=w41:T2)
            n9 = call <vilib>:"CTRE_Phoenix_MotorControl_ConfigBaseSettings.vi"("timeoutMs"=w40, "Force Write"=w38, "Base Configurables"=w41, "PhoenixMotorControlDevRef in"=w42) -> ("error out"=w37:errorcluster, "PhoenixMotorControlDevRef out"=w39:T12)  [unwired: 6 in]
          }
          frame 2 {
            n10 = Unbundle By Name(w48) -> ("forwardLimitSwitchSource"=w47:bool, "forwardLimitSwitchNormal"=w46:bool, "forwardLimitSwitchDeviceID"=w45:bool)
            n11 = Compound Arithmetic op=OR(w47, w46, w45) -> (w44:bool)
            n12 = case shown="True" w44 {
              tunnel: w53 -> [_ w63]
              tunnel: w52 -> [w55 w59]
              tunnel: [w55 w58] -> w51
              tunnel: [errorcluster {"status"=FALSE, "code"=0, "source"=""} ("error out") w57] -> w50
              tunnel: w49 -> [_ w56]
              frame False {
              }
              frame True {
                n13 = Unbundle By Name(w63) -> ("forwardLimitSwitchSource"=w62:T11, "forwardLimitSwitchNormal"=w61:T10, "forwardLimitSwitchDeviceID"=w60:i32)
                n14 = call <vilib>:"CTRE_Phoenix_MotorControl_ConfigForwardLimitSwitch.vi"("PhoenixMotorControlDevRef"=w59, "LimitSwitchSource"=w62, "NormallyOpenOrClosed"=w61, "deviceID"=w60, "timeoutMs"=w56) -> ("PhoenixMotorControlDevRef"=w58:T12, "error out"=w57:errorcluster)  [unwired: 9 in]
              }
            }
          }
          frame 3 {
            n15 = Unbundle By Name(w68) -> ("forwardLimitSwitchSource"=w67:bool, "reverseLimitSwitchNormal"=w66:bool, "reverseLimitSwitchDeviceID"=w65:bool)
            n16 = Compound Arithmetic op=OR(w67, w66, w65) -> (w64:bool)
            n17 = case shown="True" w64 {
              tunnel: w73 -> [_ w83]
              tunnel: w72 -> [w75 w79]
              tunnel: [w75 w78] -> w71
              tunnel: [errorcluster {"status"=FALSE, "code"=0, "source"=""} ("error out") w77] -> w70
              tunnel: w69 -> [_ w76]
              frame False {
              }
              frame True {
                n18 = Unbundle By Name(w83) -> ("reverseLimitSwitchSource"=w82:T11, "reverseLimitSwitchNormal"=w81:T10, "reverseLimitSwitchDeviceID"=w80:i32)
                n19 = call <vilib>:"CTRE_Phoenix_MotorControl_ConfigReverseLimitSwitch.vi"("PhoenixMotorControlDevRef"=w79, "LimitSwitchSource"=w82, "NormallyOpenOrClosed"=w81, "deviceID"=w80, "timeoutMs"=w76) -> ("PhoenixMotorControlDevRef"=w78:T12, "error out"=w77:errorcluster)  [unwired: 9 in]
              }
            }
          }
          frame 4 {
            # "Config Primary Feedback Coefficient"
            n20 = Unbundle By Name(w85) -> ("primaryPID.selectedFeedbackCoefficient"=w84:bool)
            n21 = case shown="True" w84 {
              tunnel: w90 -> [_ w99]
              tunnel: w89 -> [w92 w98]
              tunnel: [w92 w96] -> w88
              tunnel: [errorcluster {"status"=FALSE, "code"=0, "source"=""} ("error out") w95] -> w87
              tunnel: w86 -> [_ w94]
              frame False {
              }
              frame True {
                n22 = Unbundle By Name(w99) -> ("primaryPID.selectedFeedbackCoefficient"=w97:dbl)
                n23 = call <vilib>:"CTRE_Phoenix_MotorControl_ConfigSelectedFeedbackCoefficient.vi"("timoutMs"=w94, "pidIdx"=0, "coefficient"=w97, "PhoenixMotorControlDevRef"=w98) -> ("error out"=w95:errorcluster, "PhoenixMotorControlDevRef"=w96:T12)  [unwired: 6 in]
              }
            }
          }
          frame 5 {
            # "Config Primary Feedback Sensor"
            n24 = Unbundle By Name(w101) -> ("primaryPID.selectedFeedbackSensor"=w100:bool)
            n25 = case shown="True" w100 {
              tunnel: w102 -> [_ w115]
              tunnel: [w108 w114] -> w106
              tunnel: w105 -> [w108 w113]
              tunnel: w104 -> [_ w110]
              tunnel: [errorcluster {"status"=FALSE, "code"=0, "source"=""} ("error out") w109] -> w103
              frame False {
              }
              frame True {
                n26 = Unbundle By Name(w115) -> ("primaryPID.selectedFeedbackSensor"=w112:T8)
                n27 = call <vilib>:"CTRE_Phoenix_MotorControl_ConfigSelectedFeedbackSensor.vi"("timeoutMs"=w110, "pidLoopIdx"=0, "Feedback Device"=w112, "PhoenixMotorControlDevRef"=w113) -> ("error out"=w109:errorcluster, "PhoenixMotorControlDevRef"=w114:T12)  [unwired: 6 in]
              }
            }
          }
          frame 6 {
            # "Config Auxiliary Feedback Coefficient"
            n28 = Unbundle By Name(w117) -> ("auxiliaryPID.selectedFeedbackCoefficient"=w116:bool)
            n29 = case shown="True" w116 {
              tunnel: w122 -> [w124 w129]
              tunnel: [w124 w128] -> w121
              tunnel: w120 -> [_ w127]
              tunnel: [errorcluster {"status"=FALSE, "code"=0, "source"=""} ("error out") w126] -> w119
              tunnel: w118 -> [_ w125]
              frame False {
              }
              frame True {
                n30 = Unbundle By Name(w125) -> ("auxiliaryPID.selectedFeedbackCoefficient"=w131:dbl)
                n31 = call <vilib>:"CTRE_Phoenix_MotorControl_ConfigSelectedFeedbackCoefficient.vi"("timoutMs"=w127, "pidIdx"=1, "coefficient"=w131, "PhoenixMotorControlDevRef"=w129) -> ("error out"=w126:errorcluster, "PhoenixMotorControlDevRef"=w128:T12)  [unwired: 6 in]
              }
            }
          }
          frame 7 {
            # "Config Auxiliary Feedback Sensor"
            n32 = Unbundle By Name(w133) -> ("auxiliaryPID.selectedFeedbackSensor"=w132:bool)
            n33 = case shown="True" w132 {
              tunnel: w138 -> [_ w147]
              tunnel: w137 -> [_ w146]
              tunnel: [errorcluster {"status"=FALSE, "code"=0, "source"=""} ("error out") w145] -> w136
              tunnel: [w140 w144] -> w135
              tunnel: w134 -> [w140 w143]
              frame False {
              }
              frame True {
                n34 = Unbundle By Name(w147) -> ("auxiliaryPID.selectedFeedbackSensor"=w142:T8)
                n35 = call <vilib>:"CTRE_Phoenix_MotorControl_ConfigSelectedFeedbackSensor.vi"("timeoutMs"=w146, "pidLoopIdx"=1, "Feedback Device"=w142, "PhoenixMotorControlDevRef"=w143) -> ("error out"=w145:errorcluster, "PhoenixMotorControlDevRef"=w144:T12)  [unwired: 6 in]
              }
            }
          }
          frame 8 {
            # "Config Sum 0"
            n36 = Unbundle By Name(w149) -> ("sum 0 term"=w148:bool)
            n37 = case shown="True" w148 {
              tunnel: w154 -> [_ w163]
              tunnel: [w156 w162] -> w153
              tunnel: w152 -> [w156 w161]
              tunnel: w151 -> [_ w158]
              tunnel: [errorcluster {"status"=FALSE, "code"=0, "source"=""} ("error out") w157] -> w150
              frame False {
              }
              frame True {
                w159 = u16 0 items=["Sum 0 (S0)", "Sum 1 (S1)", "Difference 0 (D0)", "Difference 1 (D1)"] ("Sensor Term")
                n38 = Unbundle By Name(w163) -> ("sum 0 term"=w160:T9)
                n39 = call <vilib>:"CTRE_Phoenix_MotorControl_ConfigSensorTerm.vi"("timeoutMs"=w158, "Sensor Term"=w159, "Feedback Device"=w160, "PhoenixMotorControlDevRef"=w161) -> ("error out"=w157:errorcluster, "PhoenixMotorControlDevRef"=w162:T12)  [unwired: 6 in]
              }
            }
          }
          frame 9 {
            # "Config Sum 1"
            n40 = Unbundle By Name(w165) -> ("sum 1 term"=w164:bool)
            n41 = case shown="True" w164 {
              tunnel: w170 -> [_ w179]
              tunnel: w169 -> [w172 w178]
              tunnel: w168 -> [_ w177]
              tunnel: [w172 w176] -> w167
              tunnel: [errorcluster {"status"=FALSE, "code"=0, "source"=""} ("error out") w175] -> w166
              frame False {
              }
              frame True {
                w174 = u16 1 items=["Sum 0 (S0)", "Sum 1 (S1)", "Difference 0 (D0)", "Difference 1 (D1)"] ("Sensor Term")
                n42 = Unbundle By Name(w179) -> ("sum 1 term"=w173:T9)
                n43 = call <vilib>:"CTRE_Phoenix_MotorControl_ConfigSensorTerm.vi"("timeoutMs"=w177, "Sensor Term"=w174, "Feedback Device"=w173, "PhoenixMotorControlDevRef"=w178) -> ("error out"=w175:errorcluster, "PhoenixMotorControlDevRef"=w176:T12)  [unwired: 6 in]
              }
            }
          }
          frame 10 {
            # "Config Diff 0"
            n44 = Unbundle By Name(w181) -> ("diff 0 term"=w180:bool)
            n45 = case shown="True" w180 {
              tunnel: w186 -> [_ w195]
              tunnel: [w188 w194] -> w185
              tunnel: [errorcluster {"status"=FALSE, "code"=0, "source"=""} ("error out") w193] -> w184
              tunnel: w183 -> [_ w192]
              tunnel: w182 -> [w188 w191]
              frame False {
              }
              frame True {
                w189 = u16 2 items=["Sum 0 (S0)", "Sum 1 (S1)", "Difference 0 (D0)", "Difference 1 (D1)"] ("Sensor Term")
                n46 = Unbundle By Name(w195) -> ("diff 0 term"=w190:T9)
                n47 = call <vilib>:"CTRE_Phoenix_MotorControl_ConfigSensorTerm.vi"("timeoutMs"=w192, "Sensor Term"=w189, "Feedback Device"=w190, "PhoenixMotorControlDevRef"=w191) -> ("error out"=w193:errorcluster, "PhoenixMotorControlDevRef"=w194:T12)  [unwired: 6 in]
              }
            }
          }
          frame 11 {
            # "Config Diff 1"
            n48 = Unbundle By Name(w197) -> ("diff 1 term"=w196:bool)
            n49 = case shown="True" w196 {
              tunnel: w202 -> [_ w211]
              tunnel: w201 -> [_ w210]
              tunnel: [w204 w209] -> w200
              tunnel: w199 -> [w204 w208]
              tunnel: [errorcluster {"status"=FALSE, "code"=0, "source"=""} ("error out") w205] -> w198
              frame False {
              }
              frame True {
                w206 = u16 3 items=["Sum 0 (S0)", "Sum 1 (S1)", "Difference 0 (D0)", "Difference 1 (D1)"] ("Sensor Term")
                n50 = Unbundle By Name(w211) -> ("diff 1 term"=w207:T9)
                n51 = call <vilib>:"CTRE_Phoenix_MotorControl_ConfigSensorTerm.vi"("timeoutMs"=w210, "Sensor Term"=w206, "Feedback Device"=w207, "PhoenixMotorControlDevRef"=w208) -> ("error out"=w205:errorcluster, "PhoenixMotorControlDevRef"=w209:T12)  [unwired: 6 in]
              }
            }
          }
          frame Default {
          }
        }
      }
      n52 = Or Array Elements(Boolean array=w16) -> (logical OR=w19:bool)
      n53 = Select(t=errorcluster {"status"=TRUE, "code"=-1, "source"="Motor Controller Configure All Settings: 1 or more configs failed"} ("error out 2"), s=w19, f=errorcluster {"status"=FALSE, "code"=0, "source"=""} ("error out 2")) -> (s? t:f=w20:errorcluster)
    }
    frame Error {
    }
  }
  "PhoenixMotorControlDevRef" <- w8
  "error out" <- w10
